vi "DFD M-Band Filter Bank Decomposition with State (Array).vi"(6 "state in":cluster{"state ":dbl[]}[](array[cluster]), 8 "error in (no error)":errorcluster, 9 "init?":bool, 10 "analysis bank":T1={"mBank_Filters"=[], " mBank_#Bands"=2, "mBank_ProcMethod"=enum."General", "mBank_Coeffs"=[], "mBank_Gain"=1.0, "mBank_Type"=0} {"mBank_Type" items=["Uniform", "Non-Uniform"]; "mBank_Filters"."mMRate_SumWl" min=1 max=32 step=1; "mBank_Filters"."mMRate_InputIwl" min=1 max=32 step=1; "mBank_Filters"."mMRate_GainWl" min=1 max=32 step=1; "mBank_Filters"."mMRate_OutputWl" min=1 max=32 step=1; "mBank_Filters"."mMRate_InputWl" min=1 max=32 step=1; "mBank_Filters"."mMRate_CoefWl" min=1 max=32 step=1; "mBank_Filters"."mMRate_Mode" items=["Default"=-1, "No Rate Change"=0, "Interpolation"=1, "Decimation"=2, "Interpolated"=3, "Rational"=4]}, 11 "M bands":dbl[](array[numeric]) format="%.2f") -> (0 "error out":errorcluster, 3 "y":dbl[][](array[numeric]), 4 "state out":cluster{"state ":dbl[]}[](array[cluster]))   [LabVIEW 2017, in "NI_DigFilter_FilterBank.lvlib"]
doc: "Filters the input sequence <B>x</B> using an M-band analysis bank specified by <B>analysis bank</B>. You must specify the most recent internal input states <B>state in</B> to get the correct output. \n\n<B>state out</B> contains the most recent internal output states, which can be used as <B>state in</B> for next call to this VI if you want to process the data continuously.\n\nYou can call the VIs in <B>Filter Bank Design</B> sub-palette to design a filter bank."
uses:
  <vilib>/addons/Digital Filter Design/NI_DigFilter_FilterBank.lvlib
  <vilib>/addons/Digital Filter Design/FilterBank.llb/Object/DFD Bank Obj.ctl
  <vilib>/addons/Digital Filter Design/_Objects.llb/DFD Multirate Filter Obj.ctl
  <vilib>/addons/Digital Filter Design/_Objects.llb/DFD Multirate Mode.ctl
  <vilib>/addons/Digital Filter Design/_Objects.llb/DFD Coef Norm Type.ctl
  <vilib>/addons/Digital Filter Design/_Objects.llb/DFD Round-off Mode.ctl
  <vilib>/addons/Digital Filter Design/_Objects.llb/DFD FXP MRate Multiply Mode.ctl
  <vilib>/addons/Digital Filter Design/FilterBank.llb/Object/DFD Filter Bank Processing Method.ctl
  <vilib>/addons/Digital Filter Design/FilterBank.llb/Object/DFD Filter Bank Type.ctl
  <vilib>/addons/Digital Filter Design/NI_DigFilter_Process.lvlib
  <vilib>/addons/Digital Filter Design/NI_DigFilterLicensed.lvlib
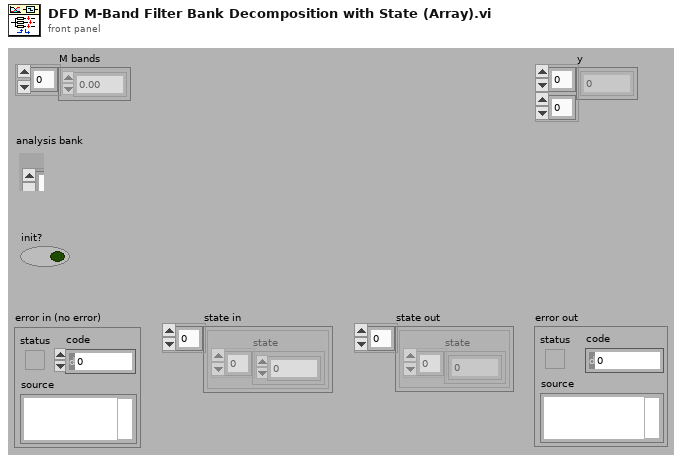
[diagram p1: front panel]
types:
  T1 = typedef "NI_DigFilter_FilterBank.lvlib/DFD Bank Obj.ctl" = cluster{"mBank_Filters":T2[], " mBank_#Bands":i32, "mBank_ProcMethod":T7, "mBank_Coeffs":dbl[], "mBank_Gain":dbl, "mBank_Type":T8}
  T2 = typedef "NI_DigFilterLicensed.lvlib/DFD Multirate Filter Obj.ctl" = cluster{"mMRate_Structure":enum16{"CIC", "FIR", "IIR", "Lattice"}, "mMRate_Mode":T3, "mMRate_Factor":i32, "mMRate_FIRParams":cluster{"mMRate_FIR_H":dbl[], "mMRate_FIR_IsNyquist?":bool, "mMRate_FIR_IsSymmetric?":bool}, "mMRate_CICParams":cluster{"mMRate_CIC_#Stage":i32, "mMRate_CIC_Lag":i32, "mMRate_CIC_Type":enum16{"Lowpass", "Highpass"}}, "mMRate_Order":i32, "mMRate_Version":string, "mMRate_Comments":string, "mMRate_RationalFactor":cluster{"mMRate_L":i32, "mMRate_M":i32}, "mMRate_Fs":dbl, "mMRate_Quantized?":bool, "mMRate_QFilterGain":dbl, "mMRate_CoefWl":i16, "mMRate_Scaling":cluster{"mMRate_ScaleByPowerOf2?":bool, "mMRate_ScaleType":T4}, "mMRate_InputWl":i16, "mMRate_OutputWl":i16, "mMRate_OutputMode":T5, "mMRate_MultMode":T6, "mMRate_BitPruning":bool, "mMRate_GainWl":i16, "mMRate_OutputFwl":i16, "mMRate_SumIwl":i16, "mMRate_InputIwl ":i16, "mMRate_SumWl":i16, "mMRate_CoefIwl":i16}
  T3 = typedef "NI_DigFilterLicensed.lvlib/DFD Multirate Mode.ctl" = i16
  T4 = typedef "NI_DigFilterLicensed.lvlib/DFD Coef Norm Type.ctl" = enum16{"No Norm", "Time Domain 1-Norm", "Time Domain 2-Norm", "Time Domain Inf-Norm"}
  T5 = typedef "NI_DigFilterLicensed.lvlib/DFD Round-off Mode.ctl" = enum16{"Nearest", "Truncation"}
  T6 = typedef "NI_DigFilterLicensed.lvlib/DFD FXP MRate Multiply Mode.ctl" = enum16{"Truncated", "Full"}
  T7 = typedef "NI_DigFilter_FilterBank.lvlib/DFD Filter Bank Processing Method.ctl" = enum16{"General", "2-Band QMF Lattice", "Cosine-Modulated"}
  T8 = typedef "NI_DigFilter_FilterBank.lvlib/DFD Filter Bank Type.ctl" = u16
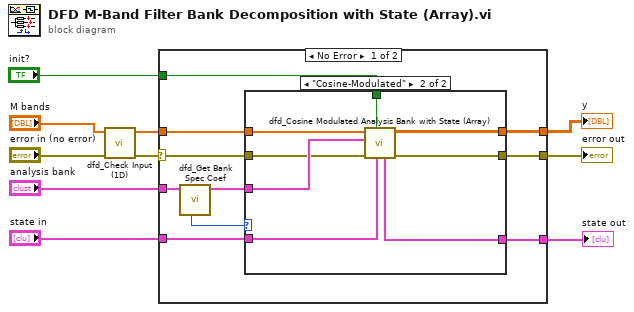
[diagram p0: block diagram]
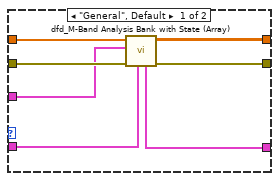
[diagram p2: hidden frame]
diagram:
  n1 = call <vilib>:"dfd_Check Input (1D).vi"("error in (no error)"="error in (no error)", "x"="M bands") -> ("error out"=w4:errorcluster, "dup x"=w2:dbl[])  [unwired: 8 in]
  n2 = case shown="No Error" w4 {
    selector: w4 -> [w15 w36]
    tunnel: "analysis bank" -> [w14 _]
    tunnel: w2 -> [w16 _]
    tunnel: "state in" -> [w20 _]
    tunnel: [w19 _] -> w6
    tunnel: [w17 w36] -> w9
    tunnel: [w18 _] -> w8
    tunnel: "init?" -> [w11 _]
    frame No Error {
      n3 = call <vilib>:"dfd_Get Bank Spec Coef.vi"("bank in"=w14) -> ("bank out"=w13:T1, "processing method"=w12:T7)  [unwired: 5 in, 4 out]
      n4 = case shown="\"Cosine-Modulated\"" w12 {
        tunnel: w16 -> [w27 w35]
        tunnel: w20 -> [w22 w32]
        tunnel: [w21 w29] -> w19
        tunnel: [w26 w34] -> w18
        tunnel: w15 -> [w25 w31]
        tunnel: [w24 w30] -> w17
        tunnel: w13 -> [w23 w33]
        tunnel: w11 -> [_ w28]
        frame "General", Default {
          n5 = call <vilib>:"dfd_M-Band Analysis Bank with State (Array).vi"("state in"=w22, "error in"=w25, "bank in"=w23, "x"=w27) -> ("error out"=w24:errorcluster, "y"=w26:dbl[][], "state out"=w21:cluster{"state ":dbl[]}[])  [unwired: 5 in]
        }
        frame "Cosine-Modulated" {
          n6 = call <vilib>:"dfd_Cosine Modulated Analysis Bank with State (Array).vi"("state in"=w32, "init?"=w28, "error in (no error)"=w31, "bank in"=w33, "x"=w35) -> ("error out"=w30:errorcluster, "y"=w34:dbl[][], "state out"=w29:cluster{"state ":dbl[]}[])  [unwired: 4 in]
        }
      }
    }
    frame Error {
    }
  }
  "error out" <- w9
  "y" <- w8
  "state out" <- w6
